vi "Max Probability.vi"(10 "A":dbl[][](array[numeric]), 11 "theta_(t-1)":dbl[](array[numeric])) -> (3 "Max Probability":dbl[](array[numeric]))   [LabVIEW 2014, in "HMM.lvlib"]
uses:
  HMM.lvlib
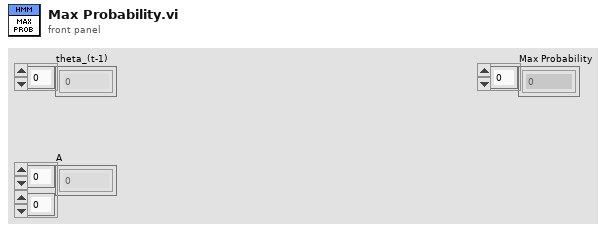
[diagram p1: front panel]
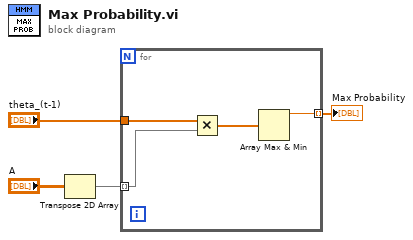
[diagram p0: block diagram]
diagram:
  n1 = Transpose 2D Array(2D array="A") -> (transposed array=w2:dbl[][])
  n2 = for {
    tunnel: w2 -> [w7] mode=indexing
    tunnel: "theta_(t-1)" -> [w8]
    tunnel: [w5] -> w1 mode=indexing
    n3 = Multiply(x=w8, y=w7) -> (x*y=w6:dbl[])
    n4 = Array Max & Min(array=w6) -> (max value=w5:dbl)  [unwired: 3 out]
  }
  "Max Probability" <- w1
